vi "ConfigureDigitizer_PedCal.vi"(6 "Clock Divisor":u32=2, 7 "Software Trig?":bool, 8 "error in (no error)":errorcluster, 9 "# Samples after Trig":u16, 10 "handle":i32, 11 "VME Base Address":u32) -> (0 "error out":errorcluster, 3 "handle out":i32, 5 "VME Base Address out":u32)   [LabVIEW 2014]
uses:
  Program Files (x86)/CAEN/Comm/labview/CAENComm.lvlib
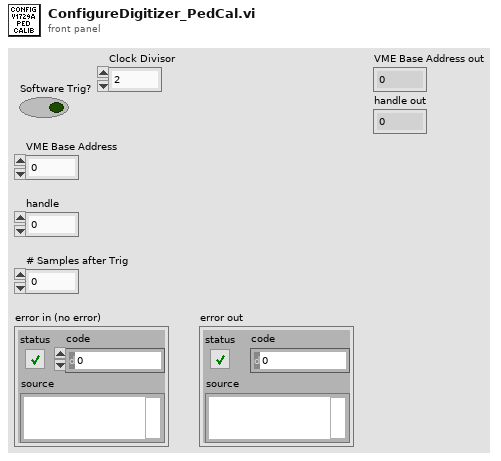
[diagram p1: front panel]
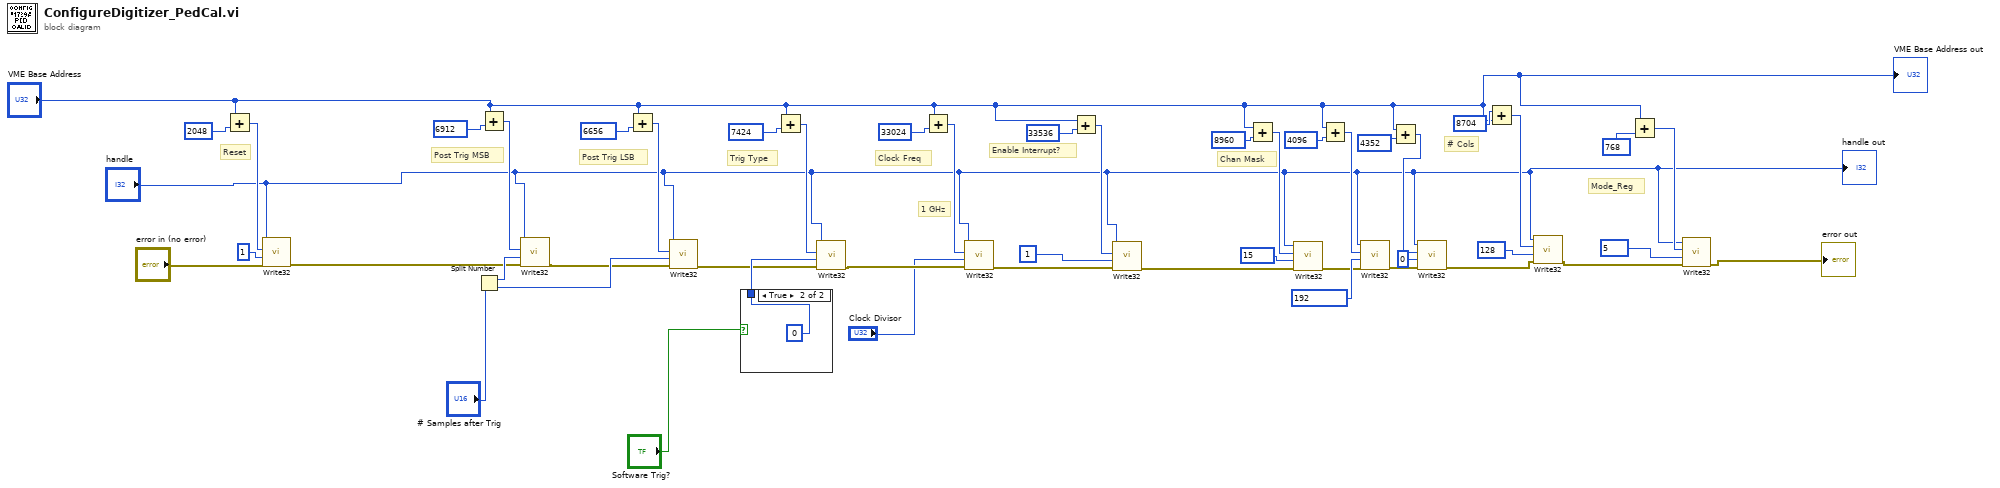
[diagram p0: block diagram]
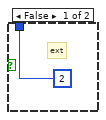
[diagram p2: hidden frame]
diagram:
  # "Mode_Reg"
  # "# Cols"
  # "Chan Mask"
  # "Enable Interrupt?"
  # "1 GHz"
  # "Clock Freq"
  # "Trig Type"
  # "Post Trig LSB"
  # "Post Trig MSB"
  # "Reset"
  n1 = Add(x="VME Base Address", y=u32 2048 ("x")) -> (x+y=w10:u32)
  n2 = call "Write32.vi"("error in (no error)"="error in (no error)", "Data"=u32 1, "Address"=w10, "handle"="handle") -> ("error out"=w8:errorcluster)  [unwired: 7 in]
  n3 = Split Number(x="# Samples after Trig") -> (hi(x)=w18:u8, lo(x)=w19:u8)
  n4 = Add(x="VME Base Address", y=u32 6912 ("x")) -> (x+y=w13:u32)
  n5 = call "Write32.vi"("error in (no error)"=w8, "Data"=w18, "Address"=w13, "handle"="handle") -> ("error out"=w17:errorcluster)  [unwired: 7 in]
  n6 = Add(x="VME Base Address", y=u32 6656 ("x")) -> (x+y=w15:u32)
  n7 = call "Write32.vi"("error in (no error)"=w17, "Data"=w19, "Address"=w15, "handle"="handle") -> ("error out"=w22:errorcluster)  [unwired: 7 in]
  n8 = case shown="True" "Software Trig?" {
    tunnel: [u8 2 ("Data") u8 0 ("Data")] -> w23
    frame False {
      # "ext"
    }
    frame True {
    }
  }
  n9 = Add(x="VME Base Address", y=u32 7424 ("x")) -> (x+y=w20:u32)
  n10 = call "Write32.vi"("error in (no error)"=w22, "Data"=w23, "Address"=w20, "handle"="handle") -> ("error out"=w27:errorcluster)  [unwired: 7 in]
  n11 = Add(x="VME Base Address", y=u32 33024 ("x")) -> (x+y=w24:u32)
  n12 = call "Write32.vi"("error in (no error)"=w27, "Data"="Clock Divisor", "Address"=w24, "handle"="handle") -> ("error out"=w31:errorcluster)  [unwired: 7 in]
  n13 = Add(x="VME Base Address", y=u32 33536 ("x")) -> (x+y=w28:u32)
  n14 = call "Write32.vi"("error in (no error)"=w31, "Data"=u8 1, "Address"=w28, "handle"="handle") -> ("error out"=w44:errorcluster)  [unwired: 7 in]
  n15 = Add(x="VME Base Address", y=u32 8960 ("x")) -> (x+y=w33:u32)
  n16 = call "Write32.vi"("error in (no error)"=w44, "Data"=u8 15, "Address"=w33, "handle"="handle") -> ("error out"=w36:errorcluster)  [unwired: 7 in]
  n17 = Add(x="VME Base Address", y=u32 4096 ("x")) -> (x+y=w38:u32)
  n18 = call "Write32.vi"("error in (no error)"=w36, "Data"=u32 192, "Address"=w38, "handle"="handle") -> ("error out"=w40:errorcluster)  [unwired: 7 in]
  n19 = Add(x="VME Base Address", y=u32 4352 ("x")) -> (x+y=w42:u32)
  n20 = call "Write32.vi"("error in (no error)"=w40, "Data"=u32 0, "Address"=w42, "handle"="handle") -> ("error out"=w47:errorcluster)  [unwired: 7 in]
  n21 = Add(x=u32 8704, y="VME Base Address") -> (x+y=w46:u32)
  n22 = call "Write32.vi"("error in (no error)"=w47, "Data"=u8 128, "Address"=w46, "handle"="handle") -> ("error out"=w4:errorcluster)  [unwired: 7 in]
  n23 = Add(x="VME Base Address", y=u32 768 ("x")) -> (x+y=w6:u32)
  n24 = call "Write32.vi"("error in (no error)"=w4, "Data"=u32 5, "Address"=w6, "handle"="handle") -> ("error out"=→"error out":errorcluster)  [unwired: 7 in]
  "VME Base Address out" <- "VME Base Address"
  "handle out" <- "handle"
